vi "Read Mid Actors.vi"(11 "Root Actors in":refnum<class "Root Actors.lvclass">) -> (2 "Mid Actors":refnum<class "Actor.lvclass">[](array[class]))   [LabVIEW 2020, in "jettl.lvlib" / "Root Actors.lvclass"]
uses:
  Root Actors.lvclass
  Actor/Actor.lvclass
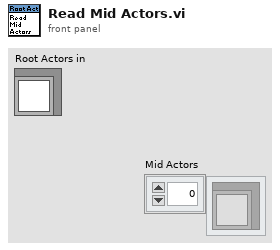
[diagram p1: front panel]
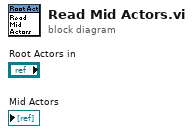
[diagram p0: block diagram]
diagram:
